vi "Actor Core.vi"(8 "error in":errorcluster, 11 "ICD System Tree View in":refnum<class "[V]System Tree View.lvclass">) -> (0 "error out":errorcluster, 3 "Actor out":refnum<class "Actor.lvclass">)   [LabVIEW 2020, in "[V]System Tree View.lvlib" / "[V]System Tree View.lvclass"]
doc: "(<B>Filename</B>: Actor Framework.lvlib:Actor.lvclass:Actor Core.vi)\n\nReceives messages to the actor, reacts to them, and initiates any error handling that may shut the actor down.\n\nDescendant classes may override this VI to append parallel tasks for the actor to complete while it handles messages. Overrides use the Call Parent Class Method node."
uses:
  [V]System Tree View.lvclass
  C:/Program Files (x86)/National Instruments/LabVIEW 2020/vi.lib/ActorFramework/Actor/Actor.lvclass
  <vilib>/ActorFramework/Actor/Actor.lvclass
  Depden On/Abstruct View/Abstruct View/Abstruct View.lvclass/Abstruct View.ctl
  [V]System Tree View.lvclass/[V]System Tree View.ctl
  <vilib>/ActorFramework/Actor/Actor.lvclass/Actor.ctl
  <vilib>/ActorFramework/Message Enqueuer/Message Enqueuer.lvclass/Message Enqueuer.ctl
  [V]System Tree View Messages/Select Channels Msg/Select Channels Msg.lvclass/Select Channels Msg.ctl
  Depden On/Abstruct View/Abstruct View/Data Accessors/Read Stop Event.vi
  <vilib>/ActorFramework/Message Enqueuer/Init from Existing Queue.vi
  <vilib>/ActorFramework/Message Enqueuer/Enqueue.vi
  <vilib>/ActorFramework/Stop Msg/Stop Msg.lvclass
  C:/Program Files (x86)/National Instruments/LabVIEW 2020/vi.lib/ActorFramework/Message/Message.lvclass
  [V]System Tree View Messages/Select Channels Msg/Select Channels Msg.lvclass
  <vilib>/ActorFramework/Message Priority Queue/Priority Enqueue.vi
  <vilib>/ActorFramework/Message Enqueuer/Message Enqueuer.lvclass
  MVVM Framework/MVVM Abstruct View/MVVM Abstruct View/MVVM Abstruct View.lvclass
panel:
  in  "Tree Multi":string[](tree)
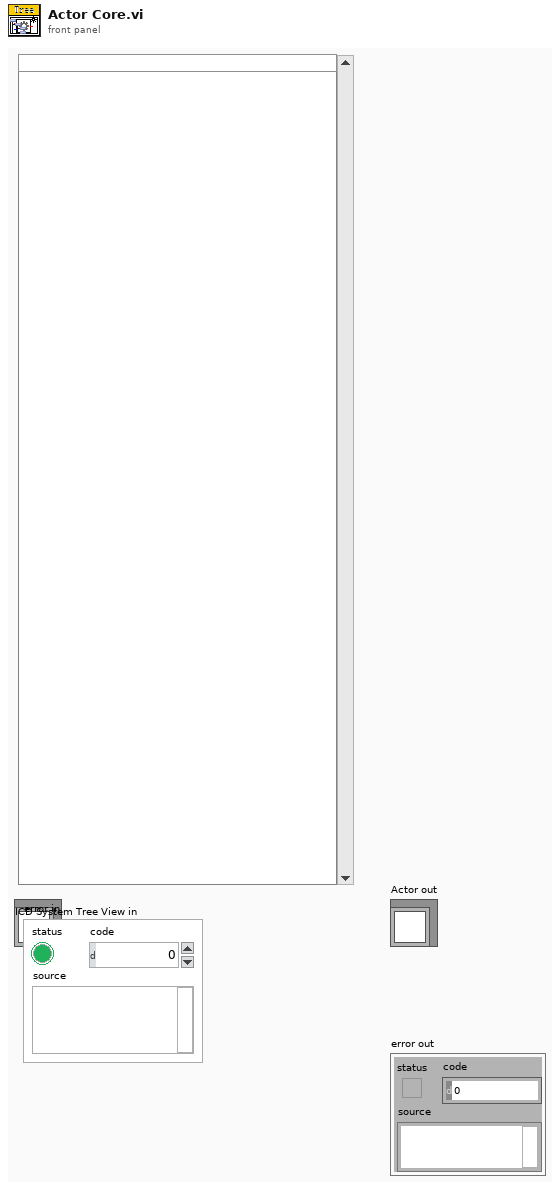
[diagram p1: front panel]
types:
  T1 = cluster{"Bold":bool, "Justification":enum16{"Left", "Center", "Right"}, "Font:Size":u32, "Font:Color":u32, "BG Color":u32}
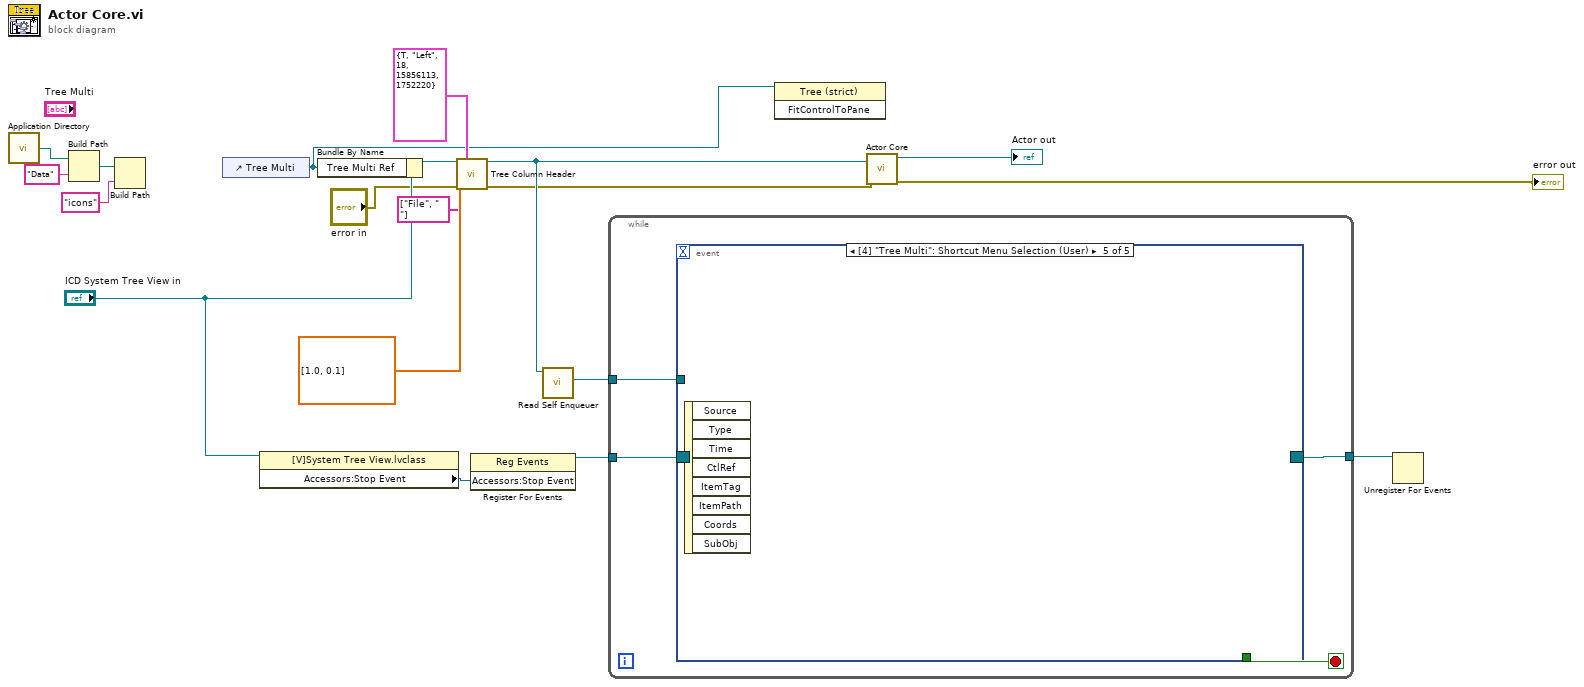
[diagram p0: block diagram]
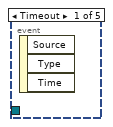
[diagram p2: hidden frame]
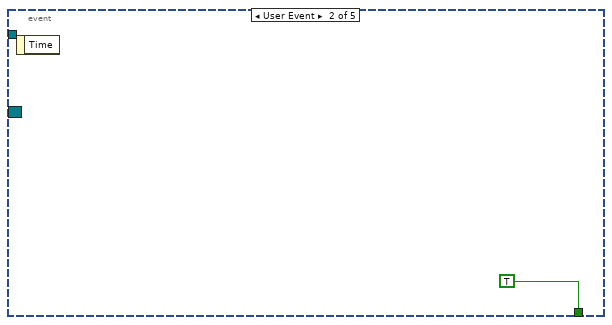
[diagram p3: hidden frame]
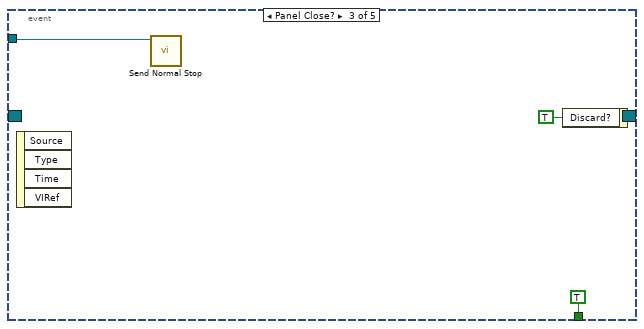
[diagram p4: hidden frame]
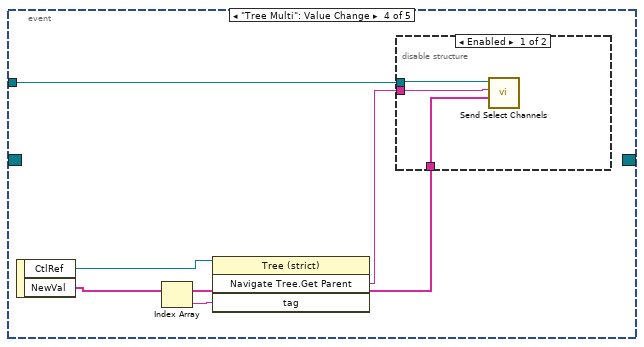
[diagram p5: hidden frame]
diagram:
  n1 = call <vilib>:"Application Directory.vi"() -> ("Application Directory"=w17:path)
  n2 = Build Path(base path=w17, name or relative path="Data") -> (appended path=w15:path)
  n3 = Build Path(base path=w15, name or relative path="icons") -> ()  [unwired: 1 out]
  n4 = control-ref of="Tree Multi"() -> (w1:refnum<vi>)
  n5 = property class="[V]System Tree View.lvclass"(reference="ICD System Tree View in") -> ("Accessors:Stop Event"=w11:refnum<user-event>)  [unwired: 1 in, 2 out]
  n6 = Bundle By Name(cluster="ICD System Tree View in", "Tree Multi Ref"=w1) -> (w13:refnum<class "[V]System Tree View.lvclass">)
  n7 = call "Tree Column Header.vi"("[V]System Tree View in"=w13, "Style"=T1 {"Bold"=TRUE, "Justification"=enum."Left", "Font:Size"=18, "Font:Color"=15856113, "BG Color"=1752220}, "Header Width Ratio"=dbl[] [1.0, 0.1], "Header Names"=string[] ["File", " "], "error in (no error)"="error in") -> ("[V]System Tree View out"=w8:refnum<class "[V]System Tree View.lvclass">, "error out"=w6:errorcluster)  [unwired: 9 in]
  n8 = register-events(w11) -> (reference out=w10:refnum<event-registration>)  [unwired: 2 in, 1 out]
  n9 = call <vilib>:"Read Self Enqueuer.vi"("Actor"=w8) -> ("Self Enqueuer"=w7:refnum<class "Message Enqueuer.lvclass">)  [unwired: 10 in]
  n10 = while {
    tunnel: [w22] -> w9
    tunnel: w10 -> [w21]
    tunnel: w7 -> [w20]
    stop <- w23 stop-if-true
    n11 = event shown="[4] \"Tree Multi\": Shortcut Menu Selection (User)" {
      selector: w21 -> [_ _ _ _ _]
      dyn-events: [_ _ _ _ _] -> w22
      timeout: _ -> [_ _ _ _ _]
      tunnel: [_ TRUE TRUE _ _] -> w23
      tunnel: w20 -> [_ _ w25 w32 _]
      event Timeout {
        n12 = event-data() -> ()  [unwired: 1 in, 3 out]
      }
      event User Event {
        n13 = event-data() -> ()  [unwired: 1 in, 1 out]
      }
      event Panel Close? {
        n14 = event-data() -> ()  [unwired: 1 in, 4 out]
        n15 = call <vilib>:"Send Normal Stop.vi"("Message Enqueuer"=w25) -> ()  [unwired: 10 in, 1 out]
        n16 = event-data("Discard?"=TRUE) -> ()  [unwired: 1 in, 1 out]
      }
      event "Tree Multi": Value Change {
        n17 = event-data() -> ("CtlRef"=w30:refnum<vi>, "NewVal"=w29:string[])  [unwired: 1 in]
        n18 = Index Array(array=w29) -> (element=w31:string)  [unwired: 1 in]
        n19 = invoke class="Tree (strict)" method="Navigate Tree.Get Parent"(reference=w30, "tag"=w31) -> ("Navigate Tree:Get Parent"=w28:string)  [unwired: 2 in, 3 out]
        n20 = disable-structure shown="Enabled" {
          disable-tunnel: w32 -> [w35 _]
          disable-tunnel: w29 -> [w33 _]
          disable-tunnel: w28 -> [w34 _]
          frame Enabled {
            n21 = call "Send Select Channels.vi"("Channel"=w33, "Table Name"=w34, "Message Enqueuer"=w35) -> ()  [unwired: 7 in, 2 out]
          }
          frame Disabled {
          }
        }
      }
      event "Tree Multi": Shortcut Menu Selection (User) {
        n22 = event-data() -> ()  [unwired: 1 in, 8 out]
      }
    }
  }
  n23 = invoke class="Tree (strict)" method="FitControlToPane"(reference=w1) -> ()  [unwired: 2 in, 3 out]
  n24 = call-parent "Actor Core.vi"("error in"=w6, "Abstruct View in"=w8) -> ("error out"=→"error out":errorcluster, "Actor out"=→"Actor out":refnum<class "Actor.lvclass">)  [unwired: 8 in]
  n25 = Unregister For Events(event registration refnum=w9) -> ()  [unwired: 1 in, 1 out]
